vi "串口基本配置对话框.vi"(11 "XML File Path":path caption="XML文件路径") -> ()   [LabVIEW 2013, in "串口配置.lvclass"]
doc: "该模板用于创建能够进行事件处理的对话框。"
uses:
  <resource>/importtools/Common/Event/NISAST Event.lvclass
panel:
  in  "串口设置":enum32{"基本", "高级"}(tab)
  in  "parity (0:none)":enum16{"None", "Odd", "Even", "Mark", "Space"}(ring) caption="奇偶（0:无）"
  in  "VISA资源名称":refnum<visa-resource-name>="COM1"
  in  "stop bits (10: 1 bit)":u16(ring)=10 caption="停止位（10: 1位）" items=["1.0"=10, "1.5"=15, "2.0"=20]
  in  "data bits (8)":u16=8 caption="数据比特(8)" min=5 max=8 step=1
  in  "baud rate (9600)":u32=9600 caption="波特率(9600)"
  in  "timeout (10sec)":u32=10000 caption="超时（10秒）"
  in  "termination char":string="\n" caption="终止符\n(0xA = '\\n' = LF)"
  in  "Enable TerminationChar (T)":bool=TRUE caption="启用终止符 (T)"
  in  "flow control (0:none)":T1(ring) caption="流控制（0:无）"
  in  "OK":bool caption="确定"
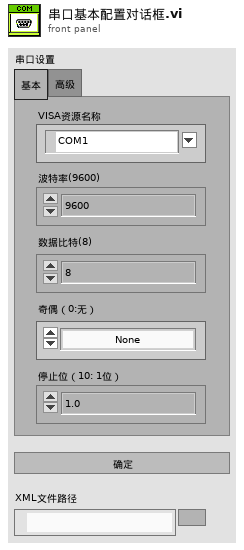
[diagram p1: front panel]
types:
  T1 = enum16{"无", "XON/XOFF", "RTS/CTS", "XON/XOFF & RTS/CTS", "DTR/DSR", "XON/XOFF & DTR/DSR"}
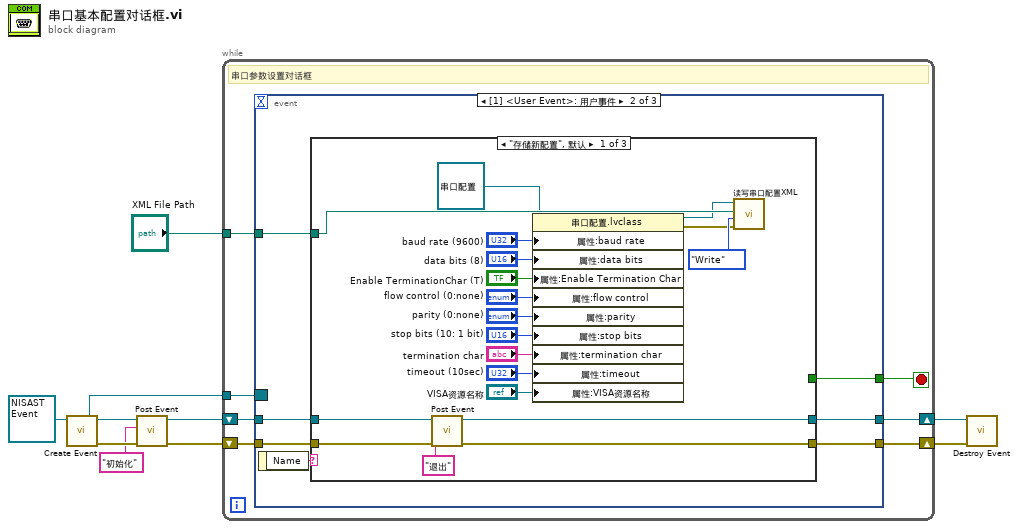
[diagram p0: block diagram]
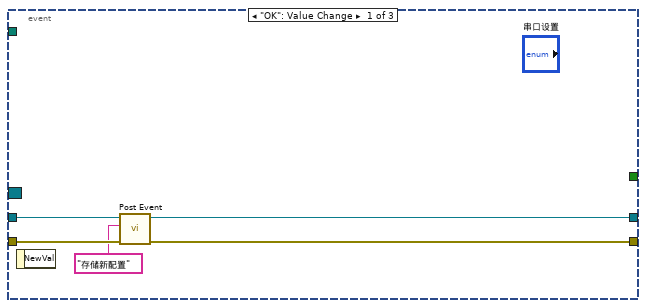
[diagram p2: hidden frame]
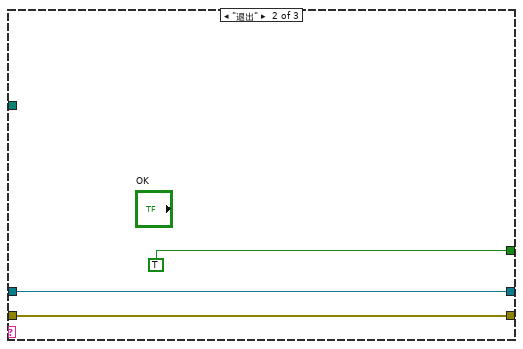
[diagram p3: hidden frame]
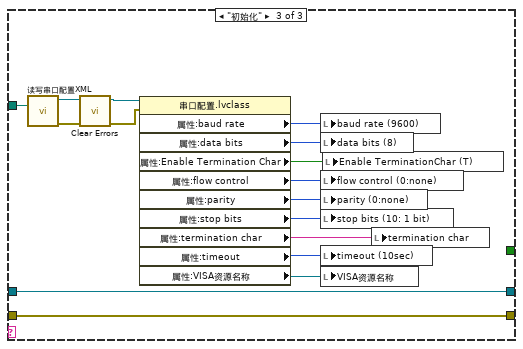
[diagram p4: hidden frame]
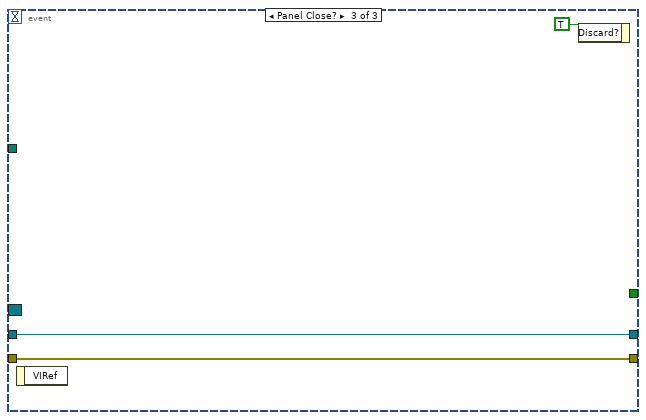
[diagram p5: hidden frame]
diagram:
  n1 = call-dynamic "Create Event.vi"("Event in"=refnum<class "NISAST Event.lvclass"> refnum) -> ("error out"=w4:errorcluster, "Event Registration Refnum"=w10:refnum<event-registration>, "Event out"=w5:refnum<class "NISAST Event.lvclass">)  [unwired: 8 in]
  n2 = call-dynamic "Post Event.vi"("error in (no error)"=w4, "Event Name"="初始化", "Event in"=w5) -> ("error out"=w1:errorcluster, "Event out"=w2:refnum<class "NISAST Event.lvclass">)  [unwired: 7 in]
  n3 = while {
    tunnel: w10 -> [w16]
    tunnel: "XML File Path" -> [w15]
    shift-right: [w13] -> w6
    shift-left: w1 -> [w14]
    shift-right: [w11] -> w7
    shift-left: w2 -> [w12]
    stop <- w17 stop-if-true
    # "串口参数设置对话框"
    n4 = event shown="[1] <User Event>: 用户事件" {
      selector: w16 -> [_ _ _]
      dyn-events: _ -> [_ _ _]
      timeout: _ -> [_ _ _]
      tunnel: [_ w27 _] -> w17
      tunnel: w15 -> [_ w28 _]
      tunnel: w14 -> [w22 w25 w68]
      tunnel: [w18 w24 w68] -> w13
      tunnel: w12 -> [w21 w26 w69]
      tunnel: [w19 w23 w69] -> w11
      event "OK": Value Change {
        n5 = event-data() -> ()  [unwired: 1 in, 1 out]
        n6 = call-dynamic "Post Event.vi"("error in (no error)"=w22, "Event Name"="存储新配置", "Event in"=w21) -> ("error out"=w18:errorcluster, "Event out"=w19:refnum<class "NISAST Event.lvclass">)  [unwired: 7 in]
      }
      event User Event {
        n7 = event-data() -> ("Name"=w29:string)  [unwired: 1 in]
        n8 = case shown="\"存储新配置\", 默认" w29 {
          tunnel: w28 -> [w48 _ w63]
          tunnel: [_ TRUE ("Cancelled?") _] -> w27
          tunnel: [w30 w50 w53] -> w23
          tunnel: w26 -> [w31 w50 w53]
          tunnel: w25 -> [w33 w49 w52]
          tunnel: [w32 w49 w52] -> w24
          frame "存储新配置", Default {
            n9 = call-dynamic "Post Event.vi"("error in (no error)"=w33, "Event Name"="退出", "Event in"=w31) -> ("error out"=w32:errorcluster, "Event out"=w30:refnum<class "NISAST Event.lvclass">)  [unwired: 7 in]
            n10 = property class="串口配置.lvclass"(reference=refnum<class "串口配置.lvclass"> refnum ("串口配置.lvclass In"), "属性:baud rate"="baud rate (9600)", "属性:data bits"="data bits (8)", "属性:Enable Termination Char"="Enable TerminationChar (T)", "属性:flow control"="flow control (0:none)", "属性:parity"="parity (0:none)", "属性:stop bits"="stop bits (10: 1 bit)", "属性:termination char"="termination char", "属性:timeout"="timeout (10sec)", "属性:VISA资源名称"="VISA资源名称") -> (reference out=w35:refnum<class "串口配置.lvclass">, error out=w36:errorcluster)  [unwired: 1 in]
            n11 = call "读写串口配置XML.vi"("error in (no error)"=w36, "模式"=enum16{"Read", "Write"}."Write", "XML File Path"=w48, "串口配置.lvclass In"=w35) -> ()  [unwired: 5 in, 2 out]
          }
          frame "退出" {
          }
          frame "初始化" {
            # "用户事件"
            n12 = call "读写串口配置XML.vi"("XML File Path"=w63) -> ("error out"=w66:errorcluster, "串口配置.Out"=w64:refnum<class "串口配置.lvclass">)  [unwired: 8 in]
            n13 = call <vilib>:"Clear Errors.vi"("error in (no error)"=w66) -> ("error out"=w65:errorcluster)  [unwired: 6 in]
            n14 = property class="串口配置.lvclass"(reference=w64, error in=w65) -> ("属性:baud rate"=w54:u32, "属性:data bits"=w55:u16, "属性:Enable Termination Char"=w56:bool, "属性:flow control"=w57:T1, "属性:parity"=w59:enum16{"None", "Odd", "Even", "Mark", "Space"}, "属性:stop bits"=w58:u16, "属性:termination char"=w60:string, "属性:timeout"=w61:u32, "属性:VISA资源名称"=w62:refnum<visa-resource-name>)  [unwired: 2 out]
            n15 = local write "baud rate (9600)"(w54) -> ()
            n16 = local write "data bits (8)"(w55) -> ()
            n17 = local write "flow control (0:none)"(w57) -> ()
            n18 = local write "parity (0:none)"(w59) -> ()
            n19 = local write "stop bits (10: 1 bit)"(w58) -> ()
            n20 = local write "timeout (10sec)"(w61) -> ()
            n21 = local write "VISA资源名称"(w62) -> ()
            n22 = local write "Enable TerminationChar (T)"(w56) -> ()
            n23 = local write "termination char"(w60) -> ()
          }
        }
      }
      event Panel Close? {
        n24 = event-data() -> ()  [unwired: 1 in, 1 out]
        n25 = event-data("Discard?"=TRUE ("放弃？")) -> ()  [unwired: 1 in, 1 out]
      }
    }
  }
  n26 = call-dynamic "Destroy Event.vi"("error in (no error)"=w6, "Event in"=w7) -> ()  [unwired: 8 in, 2 out]
